vi "step_motor_command.vi"(8 "error in":errorcluster, 9 "Ajuste?":bool=TRUE, 11 "step_motor_data":T1={"SerialPort"="", "MinTime"=0.0, "baud rate"=57600, "data bits"=8, "parity"=enum."None", "stop bits"=10, "flow control"=0, "Steps"=0, "Active"=FALSE} {"flow control" items=["None", "XON/XOFF", "RTS/CTS", "XON/XOFF & RTS/CTS", "DTR/DSR", "XON/XOFF & DTR/DSR"]; "stop bits" items=["1.0"=10, "1.5"=15, "2.0"=20]; "data bits" min=5 max=8 step=1}) -> (0 "error out":errorcluster, 2 "Respostas":string, 3 "output cluster":T1={"SerialPort"="", "MinTime"=0.0, "baud rate"=9600, "data bits"=8, "parity"=enum."None", "stop bits"=10, "flow control"=0, "Steps"=0, "Active"=FALSE} {"flow control" items=["None", "XON/XOFF", "RTS/CTS", "XON/XOFF & RTS/CTS", "DTR/DSR", "XON/XOFF & DTR/DSR"]; "stop bits" items=["1.0"=10, "1.5"=15, "2.0"=20]; "data bits" min=5 max=8 step=1})   [LabVIEW 2018]
uses:
  step_motor_data.ctl
panel:
  out "Tempo":dbl
  in  "Avançar?":bool=TRUE
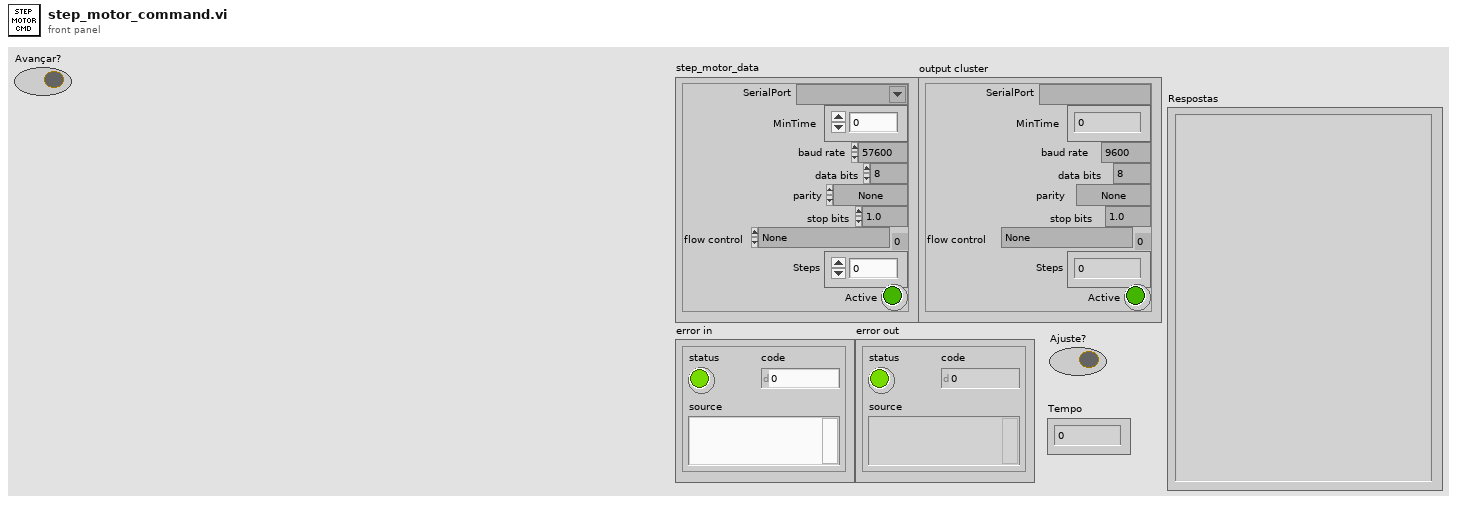
[diagram p1: front panel]
types:
  T1 = typedef "step_motor_data.ctl" = cluster{"SerialPort":refnum<visa-resource-name>, "MinTime":dbl, "baud rate":u32, "data bits":u16, "parity":enum16{"None", "Odd", "Even", "Mark", "Space"}, "stop bits":u16, "flow control":u16, "Steps":i32, "Active":bool}
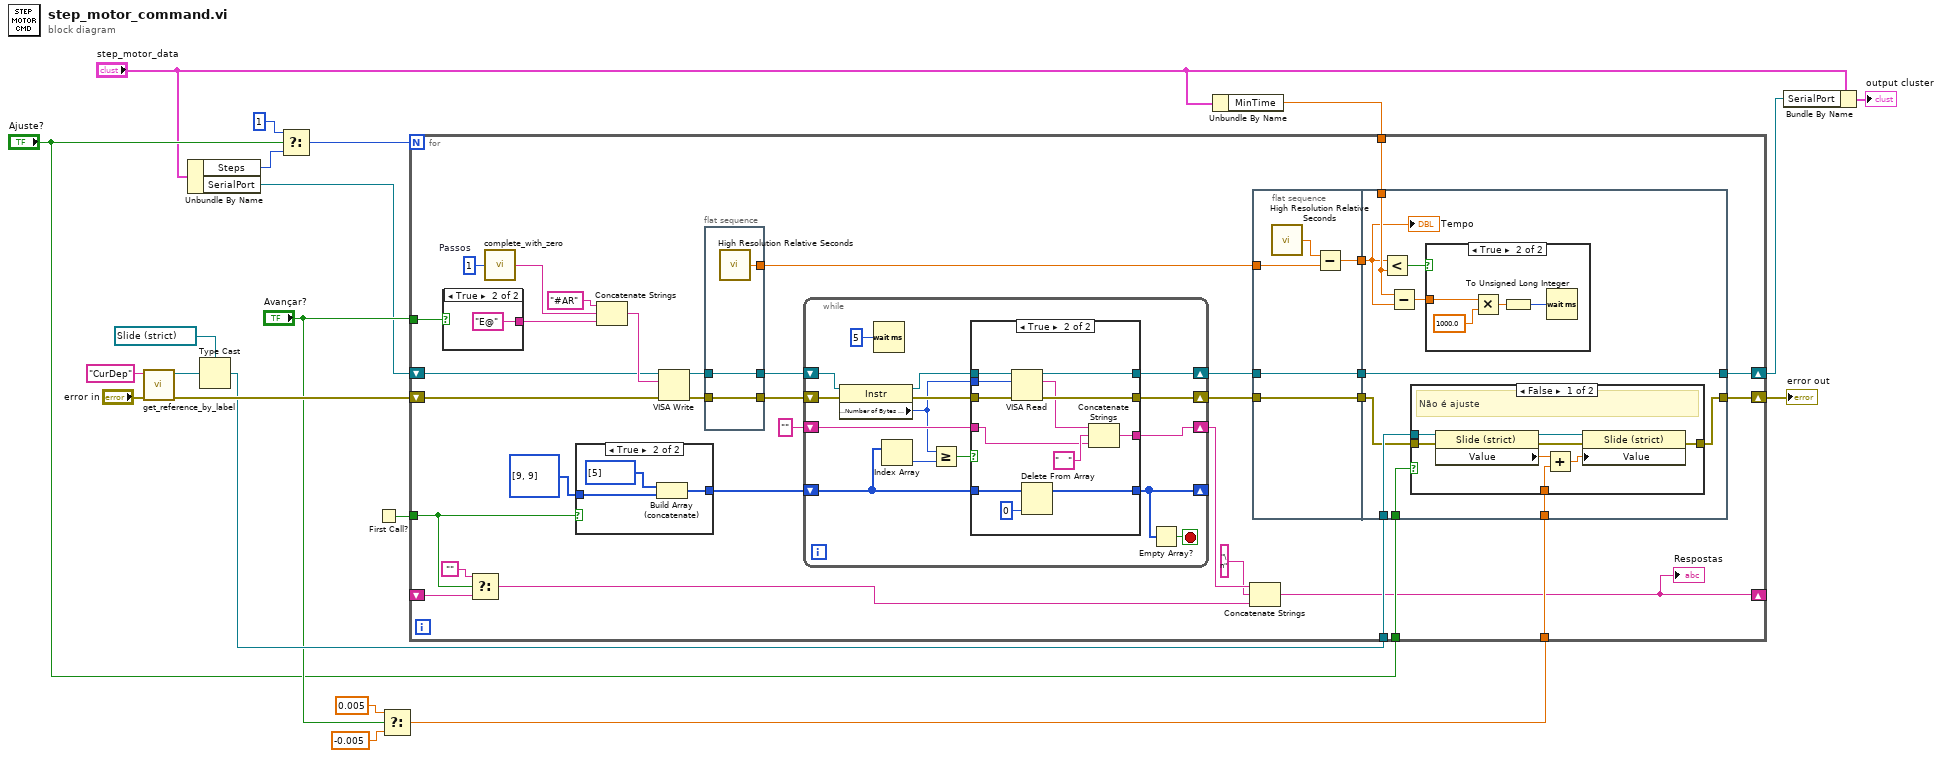
[diagram p0: block diagram]
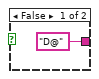
[diagram p5: hidden frame]
diagram:
  n1 = call "get_reference_by_label.vi"("error in"="error in", "Label"="CurDep") -> ("error out"=w17:errorcluster, "Ctl Refnum"=w14:refnum<vi>)  [unwired: 7 in, 1 out]
  n2 = Unbundle By Name("step_motor_data") -> ("Steps"=w3:i32, "SerialPort"=w2:refnum<visa-resource-name>)
  n3 = Type Cast(type=refnum<vi> refnum ("CurrentDepth"), x=w14) -> (*(type *) &x=w16:refnum<vi>)
  n4 = Select(t=1, s="Ajuste?", f=w3) -> (s? t:f=w5:i32)
  n5 = First Call?() -> (First Call?: T/F=w1:bool)
  n6 = Select(t=0.005, s="Avançar?", f=-0.005 ("t")) -> (s? t:f=w8:dbl)
  n7 = Unbundle By Name("step_motor_data") -> ("MinTime"=w21:dbl)
  n8 = for {
    N: w5 -> [_]
    shift-right: [w42] -> w19
    shift-left: w17 -> [w49]
    shift-right: [w37] -> w20
    shift-left: w2 -> [w39]
    tunnel: "Avançar?" -> [w36]
    tunnel: w21 -> [w34]
    tunnel: w16 -> [w33]
    tunnel: "Ajuste?" -> [w32]
    tunnel: w8 -> [w31]
    tunnel: w1 -> [w25]
    shift-right: [w22] -> _
    shift-left: _ -> [w26]
    w51 = 1  # Passos
    n9 = case shown="True" w36 {
      tunnel: ["D@" ("Command") "E@" ("Command")] -> w54
      frame False {
      }
      frame True {
      }
    }
    n10 = Select(t="", s=w25, f=w26) -> (s? t:f=w23:string)
    n11 = call "complete_with_zero.vi"("Number"=w51) -> ("StringOut"=w50:string)  [unwired: 4 in]
    n12 = case shown="True" w25 {
      tunnel: u32[] [9, 9] ("Serial Settings:Number of Bytes at Serial Port") -> [w56 w59]
      tunnel: [w56 w57] -> w29
      frame False {
      }
      frame True {
        n13 = Build Array (concatenate)(u32[] [5] ("Serial Settings:Number of Bytes at Serial Port"), w59) -> (w57:u32[])
      }
    }
    n14 = Concatenate Strings("#AR" ("Command"), w50, w54) -> (w53:string)
    n15 = VISA Write(VISA resource name=w39, write buffer=w53, error in (no error)=w49) -> (VISA resource name out=w48:refnum<visa-resource-name>, error out=w46:errorcluster)  [unwired: 1 out]
    n16 = flat-sequence {
      tunnel: w48 -> [w90]
      tunnel: [w90] -> w47
      tunnel: w46 -> [w89]
      tunnel: [w89] -> w45
      tunnel: [w88] -> w41
      frame #0 {
        n17 = call <vilib>:"High Resolution Relative Seconds.vi"() -> ("relative seconds"=w88:dbl)
      }
    }
    n18 = while {
      shift-right: [w102] -> w44
      shift-left: w45 -> [w103]
      shift-right: [w101] -> w28
      shift-left: "" -> [w100]
      shift-right: [w107] -> w43
      shift-left: w47 -> [w104]
      shift-right: [w94] -> _
      shift-left: w29 -> [w95]
      stop <- w93 stop-if-true
      n19 = property class="Instr"(reference=w104, error in=w103) -> (reference out=w106:refnum<visa-resource-name>, error out=w105:errorcluster, "Serial Settings:Number of Bytes at Serial Port"=w98:u32)
      n20 = Wait (ms)(milliseconds to wait=u32 5) -> ()  [unwired: 1 out]
      n21 = Index Array(array=w95) -> (element=w97:u32)  [unwired: 1 in]
      n22 = Greater Or Equal?(x=w98, y=w97) -> (x >= y?=w96:bool)
      n23 = case shown="True" w96 {
        tunnel: [w110 w123] -> w102
        tunnel: [w111 w122] -> w107
        tunnel: w106 -> [w111 w121]
        tunnel: w105 -> [w110 w120]
        tunnel: w98 -> [_ w117]
        tunnel: [w109 w118] -> w101
        tunnel: w100 -> [w109 w112]
        tunnel: w95 -> [w108 w116]
        tunnel: [w108 w114] -> w94
        frame False {
        }
        frame True {
          n24 = VISA Read(VISA resource name=w121, byte count=w117, error in (no error)=w120) -> (VISA resource name out=w122:refnum<visa-resource-name>, read buffer=w113:string, error out=w123:errorcluster)  [unwired: 1 out]
          n25 = Delete From Array(array=w116, index=0) -> (array with subset deleted=w114:u32[])  [unwired: 1 in, 1 out]
          n26 = Concatenate Strings(w113, "   " ("string"), w112) -> (w118:string)
        }
      }
      n27 = Empty Array?(array=w94) -> (empty?=w93:bool)
    }
    n28 = Concatenate Strings(w28, "\n" ("string"), w23) -> (w22:string)
    "Respostas" <- w22
    n29 = flat-sequence {
      tunnel: w44 -> [w64]
      tunnel: w43 -> [w61]
      tunnel: w41 -> [w62]
      tunnel: [w64] -> w40
      tunnel: [w61] -> w38
      tunnel: [w60] -> w35
      tunnel: [w66] -> w42
      tunnel: w40 -> [w68]
      tunnel: w38 -> [w74]
      tunnel: [w74] -> w37
      tunnel: w35 -> [w65]
      tunnel: w34 -> [w72]
      tunnel: w33 -> [w69]
      tunnel: w32 -> [w70]
      tunnel: w31 -> [w67]
      frame #0 {
        n30 = call <vilib>:"High Resolution Relative Seconds.vi"() -> ("relative seconds"=w63:dbl)
        n31 = Subtract(x=w63, y=w62) -> (x-y=w60:dbl)
      }
      frame #1 {
        n32 = Less?(x=w65, y=w72) -> (x < y?=w73:bool)
        n33 = Subtract(x=w72, y=w65) -> (x-y=w71:dbl)
        n34 = case shown="False" w70 {
          tunnel: w69 -> [w82 _]
          tunnel: w68 -> [w81 w83]
          tunnel: w67 -> [w79 _]
          tunnel: [w75 w83] -> w66
          frame False {
            # "Não é ajuste"
            n35 = property on="Property Node" class="Slide (strict)"(reference=w82, error in=w81) -> (reference out=w76:refnum<vi>, error out=w77:errorcluster, "Value"=w80:dbl)
            n36 = Add(x=w80, y=w79) -> (x+y=w78:dbl)
            n37 = property on="Property Node" class="Slide (strict)"(reference=w76, error in=w77, "Value"=w78) -> (error out=w75:errorcluster)  [unwired: 1 out]
          }
          frame True {
          }
        }
        n38 = case shown="True" w73 {
          tunnel: w71 -> [_ w87]
          frame False {
          }
          frame True {
            n39 = Multiply(x=w87, y=1000.0) -> (x*y=w85:dbl)
            n40 = To Unsigned Long Integer(number=w85) -> (unsigned 32bit integer=w84:u32)
            n41 = Wait (ms)(milliseconds to wait=w84) -> ()  [unwired: 1 out]
          }
        }
        "Tempo" <- w65
      }
    }
  }
  "error out" <- w19
  n42 = Bundle By Name(cluster="step_motor_data", "SerialPort"=w20) -> (→"output cluster":T1)
